vi "Write Boolean.vi"(8 "error in (no error)":errorcluster, 10 "Boolean":bool, 11 "dependencyData in":refnum<class "dependencyData.lvclass">) -> (0 "error out":errorcluster, 3 "dependencyData out":refnum<class "dependencyData.lvclass">)   [LabVIEW 2020, in "eos.lvlib" / "dependencyData.lvclass"]
uses:
  dependencyData.lvclass
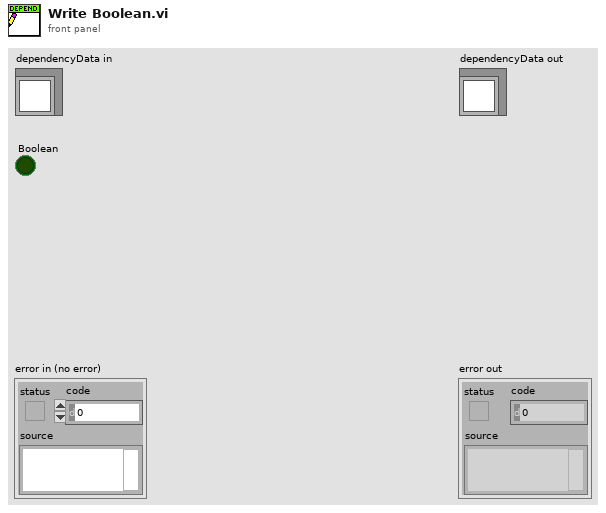
[diagram p1: front panel]
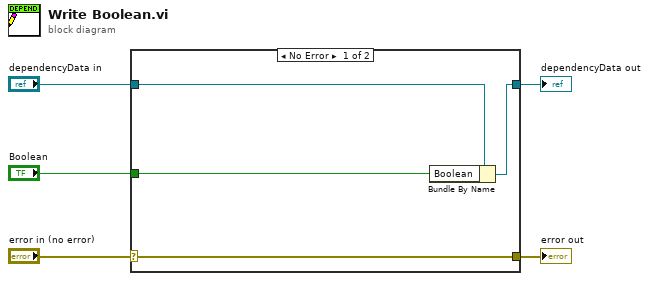
[diagram p0: block diagram]
diagram:
  n1 = case shown="No Error" "error in (no error)" {
    selector: "error in (no error)" -> [w9 w10]
    tunnel: [w9 w10] -> w4
    tunnel: [w7 w11] -> w2
    tunnel: "dependencyData in" -> [w8 w11]
    tunnel: "Boolean" -> [w6 _]
    frame No Error {
      n2 = Bundle By Name(cluster=w8, "Boolean"=w6) -> (w7:refnum<class "dependencyData.lvclass">)
    }
    frame Error {
    }
  }
  "error out" <- w4
  "dependencyData out" <- w2
